vi "BinanceAPI_emptyValueDeleter.vi"(8 "error in (no error)":errorcluster, 11 "API_TOTAL_PARAMETERS with NaN":string) -> (0 "error out":errorcluster, 3 "API_TOTAL_PARAMETERS withOUT NaN":string)   [LabVIEW 2022 SP3, in "BinanceAPI_.lvclass"]
doc: "Used only inside of BinanceAPI class. Do not use."
uses:
  src/BinanceAPI_.lvclass
  <vilib>/regexp/Match Regular Expression.xnode
panel:
  # "IN"
  # "OUT"
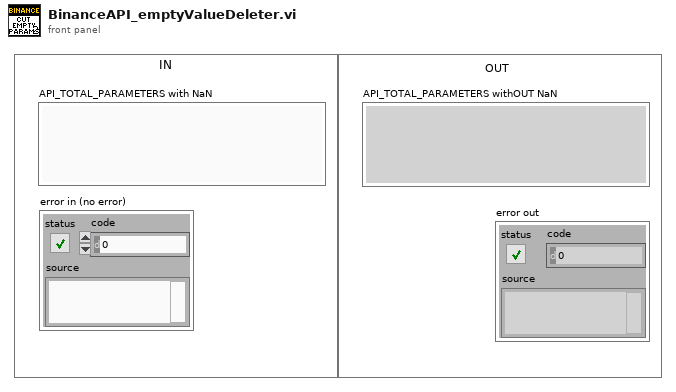
[diagram p1: front panel]
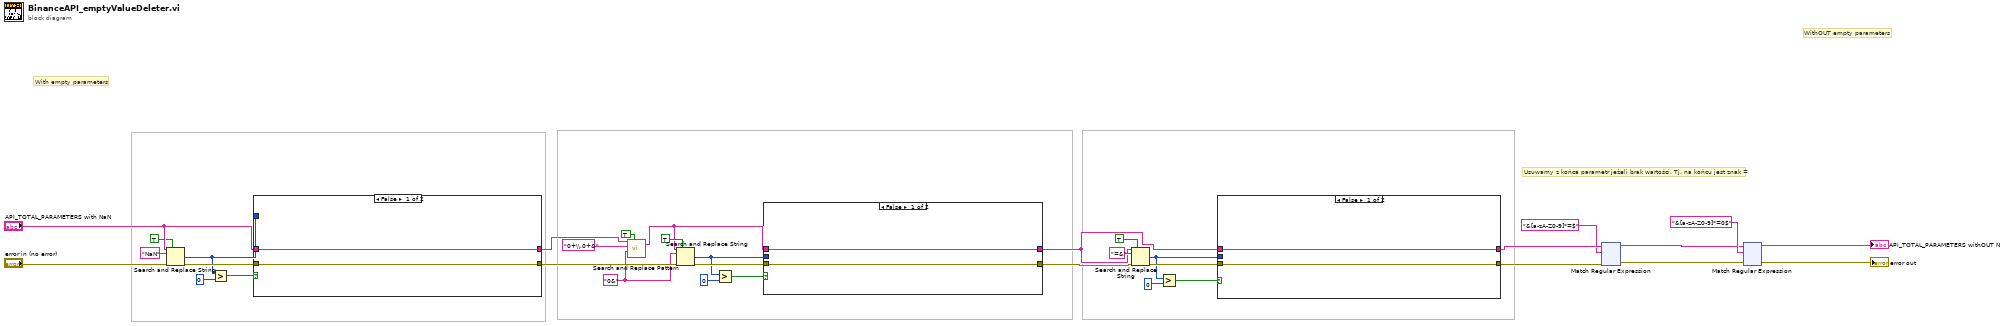
[diagram p0: block diagram]
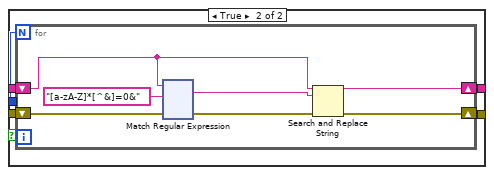
[diagram p2: hidden frame]
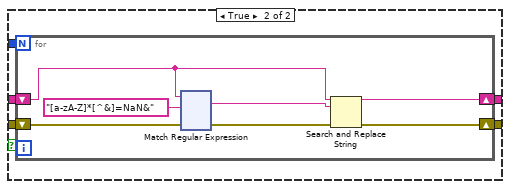
[diagram p3: hidden frame]
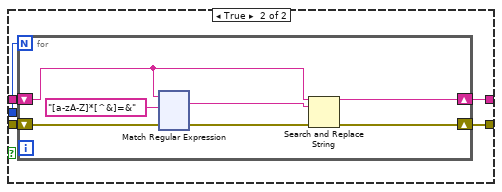
[diagram p4: hidden frame]
diagram:
  w2 = "0&" ("search string")
  # "Usuwamy z końca parametr jeżeli brak wartości. Tj. na końcu jest znak ="
  # "WithOUT empty parameters"
  # "With empty parameters"
  n1 = Search and Replace String(replace all?=TRUE ("replace all? (F)"), input string="API_TOTAL_PARAMETERS with NaN", search string="NaN", error in="error in (no error)") -> (number of replacements=w19:i32, error out=w32:errorcluster)  [unwired: 4 in, 2 out]
  n2 = Greater?(x=w19, y=0) -> (0:w17:bool)
  n3 = case shown="False" w17 {
    tunnel: "API_TOTAL_PARAMETERS with NaN" -> [w37 w42]
    tunnel: w19 -> [_ w41]
    tunnel: w32 -> [w36 w40]
    tunnel: [w36 w39] -> w28
    tunnel: [w37 w38] -> w4
    frame False {
    }
    frame True {
      n4 = for {
        N: w41 -> [_]
        shift-right: [w46] -> w38
        shift-left: w42 -> [w48]
        shift-right: [w43] -> w39
        shift-left: w40 -> [w45]
        n5 = xnode "Match Regular Expression"("input string"=w48, "regular expression"="[a-zA-Z]*[^&]=NaN&", "error in"=w45) -> ("whole match"=w47:string, "error out"=w44:errorcluster)  [unwired: 3 in, 3 out]
        n6 = Search and Replace String(input string=w48, search string=w47, error in=w44) -> (result string=w46:string, error out=w43:errorcluster)  [unwired: 5 in, 2 out]
      }
    }
  }
  n7 = call <vilib>:"Search and Replace Pattern.vi"("string"=w4, "regular expression (\"\")"="0+\\.0+&" ("search string"), "replace string (\"\")"=w2, "replace all? (F)"=TRUE) -> ("result string"=w3:string)  [unwired: 1 in, 1 out]
  n8 = Search and Replace String(replace all?=TRUE ("replace all? (F)"), input string=w3, search string=w2, error in=w28) -> (number of replacements=w15:i32, error out=w30:errorcluster)  [unwired: 4 in, 2 out]
  n9 = Greater?(x=w15, y=0) -> (0:w8:bool)
  n10 = case shown="False" w8 {
    tunnel: w30 -> [w168 w173]
    tunnel: w3 -> [w167 w172]
    tunnel: [w167 w171] -> w7
    tunnel: [w168 w170] -> w6
    tunnel: w15 -> [_ w169]
    frame False {
    }
    frame True {
      n11 = for {
        N: w169 -> [_]
        shift-right: [w177] -> w171
        shift-left: w172 -> [w179]
        shift-right: [w174] -> w170
        shift-left: w173 -> [w176]
        n12 = xnode "Match Regular Expression"("input string"=w179, "regular expression"="[a-zA-Z]*[^&]=0&", "error in"=w176) -> ("whole match"=w178:string, "error out"=w175:errorcluster)  [unwired: 3 in, 3 out]
        n13 = Search and Replace String(input string=w179, search string=w178, error in=w175) -> (result string=w177:string, error out=w174:errorcluster)  [unwired: 5 in, 2 out]
      }
    }
  }
  n14 = Search and Replace String(replace all?=TRUE ("replace all? (F)"), input string=w7, search string="=&", error in=w6) -> (number of replacements=w14:i32, error out=w25:errorcluster)  [unwired: 4 in, 2 out]
  n15 = Greater?(x=w14, y=0) -> (0:w12:bool)
  n16 = case shown="False" w12 {
    tunnel: w25 -> [w298 w304]
    tunnel: [w299 w303] -> w24
    tunnel: w7 -> [w299 w302]
    tunnel: w14 -> [_ w301]
    tunnel: [w298 w300] -> w11
    frame False {
    }
    frame True {
      n17 = for {
        N: w301 -> [_]
        shift-right: [w308] -> w303
        shift-left: w302 -> [w310]
        shift-right: [w305] -> w300
        shift-left: w304 -> [w307]
        n18 = xnode "Match Regular Expression"("input string"=w310, "regular expression"="[a-zA-Z]*[^&]=&", "error in"=w307) -> ("whole match"=w309:string, "error out"=w306:errorcluster)  [unwired: 3 in, 3 out]
        n19 = Search and Replace String(input string=w310, search string=w309, error in=w306) -> (result string=w308:string, error out=w305:errorcluster)  [unwired: 5 in, 2 out]
      }
    }
  }
  n20 = xnode "Match Regular Expression"("input string"=w24, "regular expression"="&[a-zA-Z0-9]*=$", "error in"=w11) -> ("before match"=w21:string, "error out"=w10:errorcluster)  [unwired: 3 in, 3 out]
  n21 = xnode "Match Regular Expression"("input string"=w21, "regular expression"="&[a-zA-Z0-9]*=0$", "error in"=w10) -> ("before match"=→"API_TOTAL_PARAMETERS withOUT NaN":string, "error out"=→"error out":errorcluster)  [unwired: 3 in, 3 out]
